vi "Stop Core.vi"(10 "final error code":i32, 11 "RDS Logger Actor in":refnum<class "RDS Logger Actor.lvclass">) -> (3 "RDS Logger Actor out":refnum<class "RDS Logger Actor.lvclass">)   [LabVIEW 2015, in "RDS Logger Actor.lvlib" / "RDS Logger Actor.lvclass"]
doc: "(<B>Filename</B>: Actor Framework.lvlib:Actor.lvclass:Stop Core.vi)\n\nDefines what the actor does before it stops. Use the <B>final error code</B> input to determine whether the actor shut down in response to an error.\n\nBy default, this method does nothing. A descendant class may override it to define behavior, such as shutting down any processes the actor initiated in its override of the Actor Core method."
uses:
  RDS Logger Actor.lvclass
  RDS Logger Actor.lvclass/RDS Logger Actor.ctl
  RDS Parent Actor/RDS Parent Actor/RDS Parent Actor.lvclass
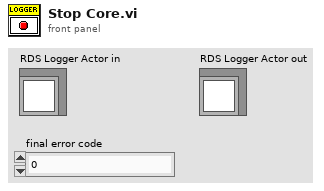
[diagram p1: front panel]
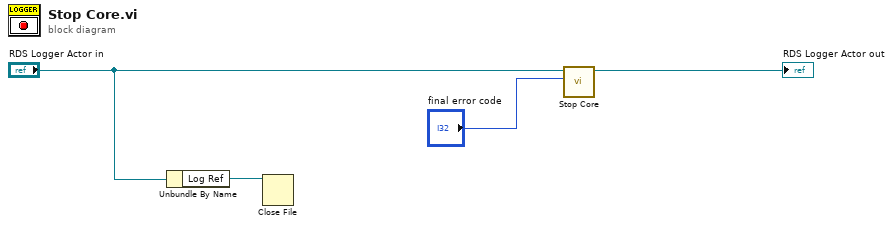
[diagram p0: block diagram]
diagram:
  n1 = Unbundle By Name("RDS Logger Actor in") -> ("Log Ref"=w1:refnum<file>)
  n2 = Close File(refnum=w1) -> ()  [unwired: 1 in, 2 out]
  n3 = call-parent "Stop Core.vi"("final error code"="final error code", "RDS Parent Actor in"="RDS Logger Actor in") -> ("RDS Parent Actor out"=→"RDS Logger Actor out":refnum<class "RDS Logger Actor.lvclass">)  [unwired: 9 in]
